vi "AprilTagCircle21h7Codes.vi"() -> (0 "Codes":i64[](array[numeric])=[8987, 11941, 13418, 17849, 31142, 32619, -19624, -6331, -423, 5485, 14347, -3925, 3460, 18230, -29582, -20720, 2364, -27724, -23293, 18063, -7881, 22421, -8382, 7197, -5668, 29613, -21153, -10960, 1994, -20690] format="%.0x", 1 "Layout":string="xxxxdddxxxxxxdddddddxxxdbbbbbbbdxxdbwwwwwbdxddbwdddwbddddbwdddwbddddbwdddwbddxdbwwwwwbdxxdbbbbbbbdxxxdddddddxxxxxxdddxxxx")   [LabVIEW 2020, in "g_ar_toolkit.feature_detection.lvlib"]
uses:
  g_ar_toolkit.feature_detection.lvlib
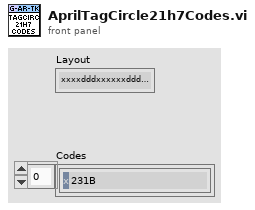
[diagram p1: front panel]
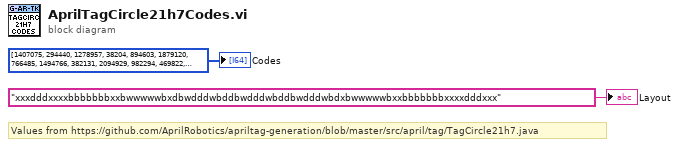
[diagram p0: block diagram]
diagram:
  # "Values from https://github.com/AprilRobotics/apriltag-generation/blob/master/src/april/tag/TagCircle21h7.java"
  "Codes" <- i64[] [1407075, 294440, 1278957, 38204, 894603, 1879120, 766485, 1494766, 382131, 2094929, 982294, 469822, 1454339, 1076822, 1676985, 786996, 402642, 2075013, 214181, 484091, 1698091, 276309, 107764, 1112792, 6994, 1566111, 946032, 971898, 825649, 85490, 657137, 938049, 1240067, 1471054, 717221, 567468, 88889, 2015715] ("Array")
  "Layout" <- "xxxdddxxxxbbbbbbbxxbwwwwwbxdbwdddwbddbwdddwbddbwdddwbdxbwwwwwbxxbbbbbbbxxxxdddxxx" ("String")
